vi "navX Example v1 (deprecated).vi"() -> ()   [LabVIEW 2015]
uses:
  navX Library v1 (deprecated)/COMMON/TypeDefs/Value TypeDefs/navX Update Rate.ctl
  navX Library v1 (deprecated)/COMMON/TypeDefs/Data TypeDefs/navX Vector Data.ctl
  navX Library v1 (deprecated)/COMMON/TypeDefs/Data TypeDefs/navX YPRH Data.ctl
  navX Library v1 (deprecated)/COMMON/TypeDefs/Data TypeDefs/navX Quaternion Data.ctl
  navX Library v1 (deprecated)/COMMON/TypeDefs/Data TypeDefs/navX Status Data.ctl
  navX Library v1 (deprecated)/COMMON/TypeDefs/Value TypeDefs/navX NAVX_OP_STATUS.ctl
  navX Library v1 (deprecated)/COMMON/TypeDefs/Value TypeDefs/navX NAVX_CAL_STATUS.ctl
  navX Library v1 (deprecated)/COMMON/TypeDefs/Value TypeDefs/navX NAVX_SELFTEST_STATUS.ctl
  navX Library v1 (deprecated)/COMMON/TypeDefs/Value TypeDefs/navX NAVX_SENSOR_STATUS.ctl
  navX Library v1 (deprecated)/COMMON/TypeDefs/Value TypeDefs/navX Interface Protocol.ctl
  navX Library v1 (deprecated)/COMMON/TypeDefs/Data TypeDefs/navX Board Information.ctl
  navX Library v1 (deprecated)/COMMON/TypeDefs/Value TypeDefs/navX NAVX_BOARD_CAPABILITY.ctl
  navX Library v1 (deprecated)/COMMON/TypeDefs/Value TypeDefs/navX NAVX_BOARD_YAW_AXIS.ctl
  navX Library v1 (deprecated)/COMMON/TypeDefs/Value TypeDefs/navX Serial Mode.ctl
  _NI WPI Serial USB/WPI_SerialPort_USB.ctl
  <vilib>/Platform/TimedLoop/XDataNode/timing_clust.ctl
  <vilib>/Platform/TimedLoop/XDataNode/nitl_modes.ctl
  <vilib>/Platform/TimedLoop/XDataNode/wakeup.ctl
  <vilib>/platform/TimedLoop/XDataNode/XDataNode.xnode
  navX Library v1 (deprecated)/navX Library v1 (deprecated).lvlib
  <vilib>/Platform/TimedLoop/XDataNode/XDNodeRunTimeDep.lvlib
  _NI WPI Serial USB/_NI WPI Serial USB.lvlib
panel:
  in  "Serial Port":T1
  in  "Nav6Mode (YPR)":T2
  out "Reboot Detected":bool
  out "CRC Err Count":i32
  out "Board Information":T3
  in  "ZeroYaw":bool
  out "Velocity":T6
  out "Displacement":T6
  in  "Reset(F)":bool
  out "Timestamp":u32
  out "Fused Heading":dbl(knob) scale=0.0..360.0
  out "MPU Temperature (Centigrade)":dbl(slide) scale=20.0..40.0
  in  "navX Interface Protocol":T7
  out "Status":T8={"Update Rate Hz"=0, "Accelerometer Full-Scale Range"=0, "Gyro Full-Scale Range"=0, "NAVX_OP_STATUS"=0, "NAVX_CAL_STATUS"=0, "NAVX_SELFTEST_STATUS"=80, "NAVX_SENSOR_STATUS"={"MOVING"=FALSE, "YAW_STABLE"=FALSE, "MAG_DISTURBANCE"=FALSE, "ALTITUDE_VALID"=FALSE, "SEALEVEL_PRESS_SET"=FALSE, "FUSED_HEADING_VALID"=FALSE}} {"NAVX_OP_STATUS" items=["INITIALIZING", "SELFTEST_IN_PROGRESS", "ERROR", "IMU_AUTOCAL_IN_PROGRESS", "NORMAL"]; "NAVX_CAL_STATUS" items=["IMU_CAL_STATE_MASK"=3, "IMU_CAL_INPROGRESS"=0, "IMU_CAL_ACCUMULATE"=1, "IMU_CAL_COMPLETE"=2, "MAG_CAL_COMPLETE"=4, "BARO_CAL_COMPLETE"=8]; "NAVX_SELFTEST_STATUS" items=["COMPLETE"=80, "GYRO_PASSED"=1, "ACCEL_PASSED"=2, "MAG_PASSED"=4, "BARO_PASSED"=8]}
  out "RawMag":T6
  out "RawGyro":T6
  out "RawAccel":T6
  out "Quaternion":T13
  out "YPRH":T14
  out "Acceleration":T6
  out "Valid?":bool
  in  "stop":bool
  out "Opened":bool
  in  "Update Rate (4Hz-60Hz)":T15=40 min=4 max=60 step=1
  # "navX"
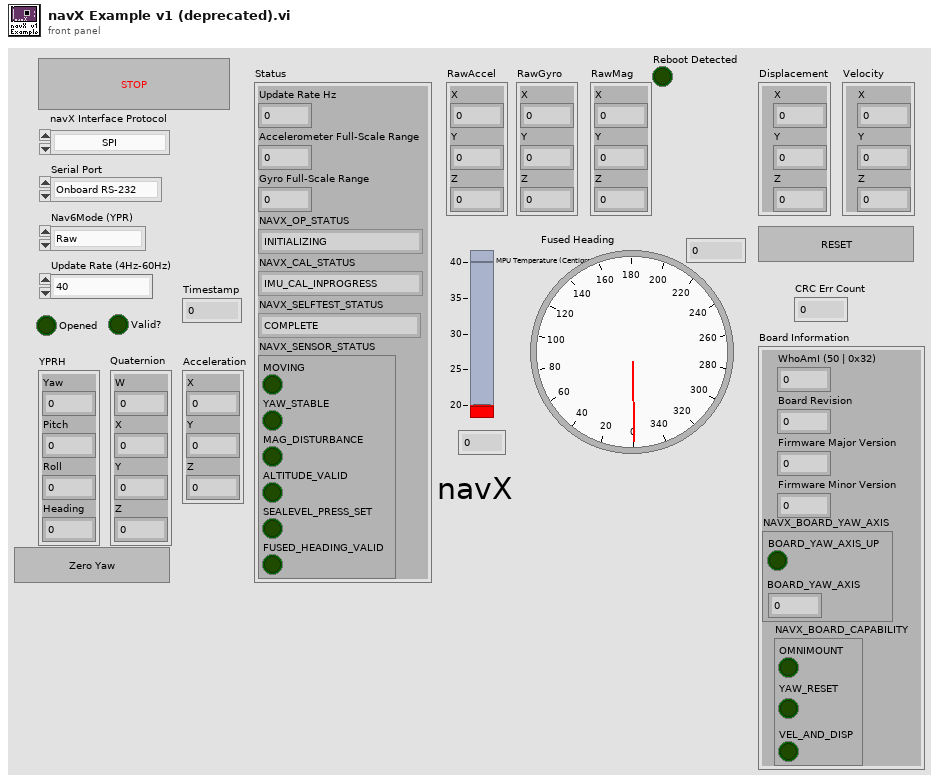
[diagram p1: front panel]
types:
  T1 = typedef "_NI WPI Serial USB.lvlib/WPI_SerialPort_USB.ctl" = enum16{"Onboard RS-232", "MXP TTL", "USB"}
  T2 = typedef "navX Library v1 (deprecated).lvlib/navX Serial Mode.ctl" = enum16{"Raw", "Processed"}
  T3 = typedef "navX Library v1 (deprecated).lvlib/navX Board Information.ctl" = cluster{"WhoAmI (50 | 0x32)":u8, "Board Revision":u8, "Firmware Major Version":u8, "Firmware Minor Version":u8, "NAVX_BOARD_CAPABILITY":T4, "NAVX_BOARD_YAW_AXIS":T5}
  T4 = typedef "navX Library v1 (deprecated).lvlib/navX NAVX_BOARD_CAPABILITY.ctl" = cluster{"OMNIMOUNT":bool, "YAW_RESET":bool, "VEL_AND_DISP":bool}
  T5 = typedef "navX Library v1 (deprecated).lvlib/navX NAVX_BOARD_YAW_AXIS.ctl" = cluster{"BOARD_YAW_AXIS_UP":bool, "BOARD_YAW_AXIS":u8}
  T6 = typedef "navX Library v1 (deprecated).lvlib/navX Vector Data.ctl" = cluster{"X":dbl, "Y":dbl, "Z":dbl}
  T7 = typedef "navX Library v1 (deprecated).lvlib/navX Interface Protocol.ctl" = enum16{"SPI", "I2C", "SERIAL"}
  T8 = typedef "navX Library v1 (deprecated).lvlib/navX Status Data.ctl" = cluster{"Update Rate Hz":u8, "Accelerometer Full-Scale Range":u8, "Gyro Full-Scale Range":u16, "NAVX_OP_STATUS":T9, "NAVX_CAL_STATUS":T10, "NAVX_SELFTEST_STATUS":T11, "NAVX_SENSOR_STATUS":T12}
  T9 = typedef "navX Library v1 (deprecated).lvlib/navX NAVX_OP_STATUS.ctl" = u8
  T10 = typedef "navX Library v1 (deprecated).lvlib/navX NAVX_CAL_STATUS.ctl" = u8
  T11 = typedef "navX Library v1 (deprecated).lvlib/navX NAVX_SELFTEST_STATUS.ctl" = u8
  T12 = typedef "navX Library v1 (deprecated).lvlib/navX NAVX_SENSOR_STATUS.ctl" = cluster{"MOVING":bool, "YAW_STABLE":bool, "MAG_DISTURBANCE":bool, "ALTITUDE_VALID":bool, "SEALEVEL_PRESS_SET":bool, "FUSED_HEADING_VALID":bool}
  T13 = typedef "navX Library v1 (deprecated).lvlib/navX Quaternion Data.ctl" = cluster{"W":dbl, "X":dbl, "Y":dbl, "Z":dbl}
  T14 = typedef "navX Library v1 (deprecated).lvlib/navX YPRH Data.ctl" = cluster{"Yaw":dbl, "Pitch":dbl, "Roll":dbl, "Heading":dbl}
  T15 = typedef "navX Library v1 (deprecated).lvlib/navX Update Rate.ctl" = u8
  T16 = typedef "navX Library v1 (deprecated).lvlib/navX Device TypeDef.ctl" = cluster{"navX Interface Protocol":T7, "navX Interface Protocol TypeDefs":cluster{"SPIDevRef":T17, "I2CDevRef":T19, "SerialPortRef":T21}, "navX System Information":cluster{"Board Information":T3, "Status":T8, "Offsets":T22, "LastSampleTimestamp":dbl, "LastSampleValid":bool}, "navX Common Information":cluster{"Update Rate (4Hz-60Hz)":T15, "refnum name":string, "error":errorcluster, "LastFPGATimestamp":dbl, "Reboot Detected":bool}, "Serial Protocol Extra":cluster{"Loop VI Refnum":refnum<vi>, "Nav6Mode (YPR)":T2}}
  T17 = typedef "WPI_SPIDevRef.ctl" = cluster{"DevStatus":errorcluster, "Handle":i32, "SPI Bus":T18}
  T18 = typedef "spi_bus.ctl" = enum16{"SPI On-Board, CS0", "SPI On-Board, CS1", "SPI On-Board, CS2", "SPI On-Board, CS3", "SPI MXP", "Invalid"}
  T19 = typedef "WPI_I2CDevRef.ctl" = cluster{"DevStatus":errorcluster, "Device Address":u8, "Handle":i32, "I2C Bus":T20}
  T20 = typedef "i2c_bus.ctl" = enum16{"I2C On-Board", "I2C MXP", "Invalid"}
  T21 = typedef "WPI_SerialPortRef.ctl" = cluster{"DevStatus":errorcluster, "Serial Port Name":refnum<visa-resource-name>}
  T22 = typedef "navX Library v1 (deprecated).lvlib/navX Offsets Data.ctl" = cluster{"Yaw":dbl, "Quat W":dbl, "Quat X":dbl, "Quat Y":dbl, "Quat Z":dbl}
  T23 = typedef "XDNodeRunTimeDep.lvlib/timing_clust.ctl" = cluster{"Expected End [f-1]":u64, "Actual End [f-1]":u64, "Finished Late? [f-1]":bool, "Expected End [i-1]":u64, "Actual End [i-1]":u64, "Finished Late? [i-1]":bool, "Expected Start [i]":u64, "Actual Start [i]":u64, "Expected Start [f]":u64, "Actual Start [f]":u64, "Source Name":string, "Structure Name":string, "Period":i64, "Deadline":i64, "Offset":i64, "Start":i64, "Priority":i32, "Timeout":i32, "Mode":T24, "Wakeup Reason":T25, "Error":errorcluster, "Source Type":string, "Secondary Source Type":string, "Global End Time":u64, "Global Start Time":u64, "Frame Duration":u64, "Iteration Duration":u64, "Assigned CPU":i32, "I/O Scan Engine Mode":u32}
  T24 = typedef "XDNodeRunTimeDep.lvlib/nitl_modes.ctl" = enum32{"No Change", "Process missed periods, maintain original phase", "Discard missed periods, maintain original phase", "Process missed periods, ignore original phase", "Discard missed periods, ignore original phase"}
  T25 = typedef "XDNodeRunTimeDep.lvlib/wakeup.ctl" = enum32{"Normal", "Aborted", "Asynchronous wakeup", "Timing source error", "Timed loop error", "Timeout"}
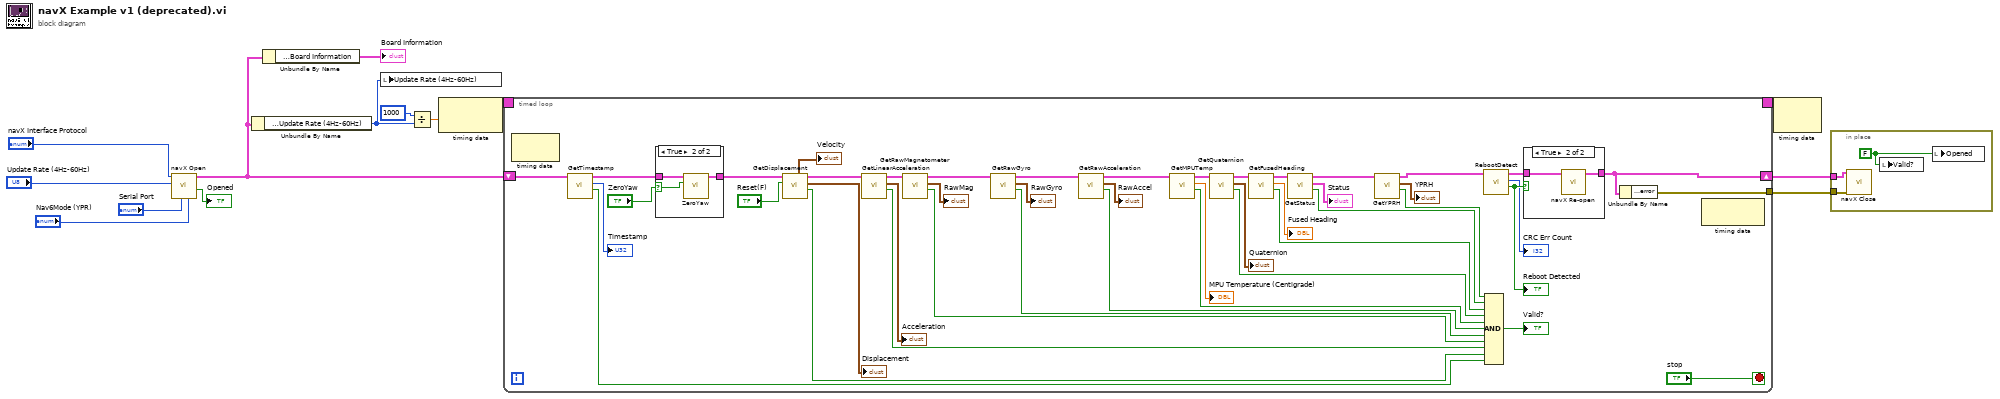
[diagram p0: block diagram]
diagram:
  n1 = call "navX Open.vi"("Nav6Mode (YPR)"="Nav6Mode (YPR)", "Serial Port"="Serial Port", "Update Rate (4Hz-60Hz)"="Update Rate (4Hz-60Hz)", "navX Interface Protocol"="navX Interface Protocol") -> ("Opened?"=→"Opened":bool, "navX Device TypeDef"=w5:T16)  [unwired: 5 in, 1 out]
  n2 = Unbundle By Name(w5) -> ("navX Common Information.Update Rate (4Hz-60Hz)"=w10:T15)
  n3 = Unbundle By Name(w5) -> ("navX System Information.Board Information"=→"Board Information":T3)
  n4 = local write "Update Rate (4Hz-60Hz)"(w10) -> ()
  n5 = Divide(x=1000, y=w10) -> (x/y=w7:dbl)
  n6 = node-c288(w7) -> (w9:T23)
  n7 = timed-loop {
    timing: w9 -> [_]
    timing-out: [_] -> w8
    tunnel: [w56] -> w6
    shift-right: [w16] -> w3
    shift-left: w5 -> [w15]
    stop <- "stop" stop-if-true
    n8 = node-c288() -> ()  [unwired: 1 in, 1 out]
    n9 = call "GetTimestamp.vi"("navX Device TypeDef"=w15) -> ("Valid?"=w27:bool, "Timestamp"=→"Timestamp":u32, "navX Device TypeDef"=w24:T16)  [unwired: 8 in]
    n10 = case shown="True" "ZeroYaw" {
      selector: "ZeroYaw" -> [_ w64]
      tunnel: w24 -> [w63 w66]
      tunnel: [w63 w65] -> w23
      frame False {
      }
      frame True {
        n11 = call "ZeroYaw.vi"("Reset(F)"=w64, "navX Device TypeDef"=w66) -> ("navX Device TypeDef"=w65:T16)  [unwired: 8 in, 1 out]
      }
    }
    n12 = call "GetDisplacement.vi"("Reset(F)"="Reset(F)", "navX Device TypeDef"=w23) -> ("Valid?"=w26:bool, "Displacement"=→"Displacement":T6, "navX Device TypeDef 2"=w30:T16, "Velocity"=→"Velocity":T6)  [unwired: 6 in]
    n13 = call "GetLinearAcceleration.vi"("navX Device TypeDef"=w30) -> ("Valid?"=w33:bool, "Linear Acceleration"=→"Acceleration":T6, "navX Device TypeDef"=w35:T16)  [unwired: 8 in]
    n14 = call "GetRawMagnetometer.vi"("navX Device TypeDef"=w35) -> ("Valid?"=w36:bool, "Raw Magnetometer"=→"RawMag":T6, "navX Device TypeDef"=w38:T16)  [unwired: 8 in]
    n15 = call "GetRawGyro.vi"("navX Device TypeDef"=w38) -> ("Valid?"=w39:bool, "Raw Gyro"=→"RawGyro":T6, "navX Device TypeDef"=w41:T16)  [unwired: 8 in]
    n16 = call "GetRawAcceleration.vi"("navX Device TypeDef"=w41) -> ("Valid?"=w42:bool, "Raw Acceleration"=→"RawAccel":T6, "navX Device TypeDef"=w44:T16)  [unwired: 8 in]
    n17 = call "GetMPUTemp.vi"("navX Device TypeDef"=w44) -> ("Valid?"=w45:bool, "MPU Temperature (Centigrade)"=→"MPU Temperature (Centigrade)":dbl, "navX Device TypeDef"=w47:T16)  [unwired: 8 in]
    n18 = call "GetQuaternion.vi"("navX Device TypeDef"=w47) -> ("Valid?"=w49:bool, "Quaternion"=→"Quaternion":T13, "navX Device TypeDef"=w50:T16)  [unwired: 8 in]
    n19 = call "GetFusedHeading.vi"("navX Device TypeDef"=w50) -> ("Valid?"=w51:bool, "Fused Heading"=→"Fused Heading":dbl, "navX Device TypeDef"=w52:T16)  [unwired: 8 in]
    n20 = call "GetStatus.vi"("navX Device TypeDef"=w52) -> ("Valid?"=w53:bool, "Status"=→"Status":T8, "navX Device TypeDef"=w55:T16)  [unwired: 8 in]
    n21 = call "GetYPRH.vi"("navX Device TypeDef"=w55) -> ("Valid?"=w58:bool, "YPRH"=→"YPRH":T14, "navX Device TypeDef"=w20:T16)  [unwired: 8 in]
    n22 = call "RebootDetect.vi"("navX Device TypeDef"=w20) -> ("Reboot Detected"=w19:bool, "Error Count"=→"CRC Err Count":i32, "navX Device TypeDef"=w18:T16)  [unwired: 8 in]
    "Reboot Detected" <- w19
    n23 = Compound Arithmetic op=AND(w58, w53, w51, w49, w45, w42, w39, w36, w33, w26, w27) -> (→"Valid?":bool)
    n24 = case shown="True" w19 {
      tunnel: w18 -> [w60 w62]
      tunnel: [w60 w61] -> w16
      frame False {
      }
      frame True {
        n25 = call "navX Re-open.vi"("navX Device TypeDef"=w62) -> ("navX Device TypeDef"=w61:T16)  [unwired: 8 in, 2 out]
      }
    }
    n26 = Unbundle By Name(w16) -> ("navX Common Information.error"=w56:errorcluster)
    n27 = node-c288() -> ()  [unwired: 1 in, 1 out]
  }
  n28 = node-c288(w8) -> ()  [unwired: 1 out]
  n29 = in-place {
    in-place-border: w3 -> [w71]
    in-place-border: w6 -> [w70]
    w69 = FALSE ("Valid?")
    n30 = call "navX Close.vi"("error in (no error)"=w70, "navX Device TypeDef"=w71) -> ()  [unwired: 9 in, 1 out]
    n31 = local write "Valid?"(w69) -> ()
    n32 = local write "Opened"(w69) -> ()
  }
